vi "dvp Vi Get Soft Trigger Loop.vi"(10 "pSoftTriggerLoop":dbl, 11 "handle":u32) -> (2 "pSoftTriggerLoop out":dbl, 3 "function return":u32(ring))   [LabVIEW 2018, in "LabViewDVPCamera.lvlib"]
doc: "LabviewDvp2Api dvpStatus dvpViGetSoftTriggerLoop(dvpHandle handle, double *pSoftTriggerLoop);"
uses:
  LabViewDVPCamera.lvlib
  LabViewDVPCamera/LabViewDVPCamera.dll
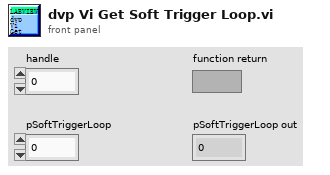
[diagram p1: front panel]
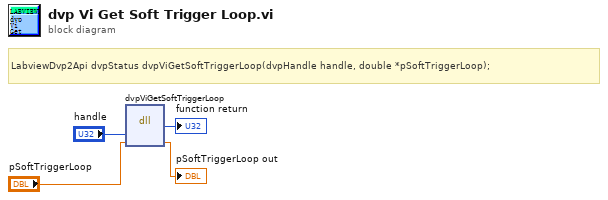
[diagram p0: block diagram]
diagram:
  # "LabviewDvp2Api dvpStatus dvpViGetSoftTriggerLoop(dvpHandle handle, double *pSoftTriggerLoop);"
  n1 = dll-call lib="C:/Program Files (x86)/DVP2 Labview cn 64/Sample/LabViewDVPCamera/LabViewDVPCamera.*" fn="dvpViGetSoftTriggerLoop"("handle"="handle", "pSoftTriggerLoop"="pSoftTriggerLoop") -> (→"function return":u32, "pSoftTriggerLoop"=→"pSoftTriggerLoop out":dbl)  [unwired: 4 in, 2 out]
